vi "CANOpen Refnum to References.vi"(8 "error in (no error)":errorcluster, 11 "CAN Session In":T4) -> (0 "error out":errorcluster, 1 "kill process notifier array":T3, 2 "Write Queue":T1, 3 "Read Queue Array":T1[](array[typedef]), 4 "New Frame Notifier":refnum<notifier>, 5 "CAN Session Queue":T2)   [LabVIEW 2016]
doc: "Extracts the read/write queue references from the CANOpen session refnum."
uses:
  Typedefs/CAN Refnum.ctl
  Typedefs/CAN Session Pointer.ctl
  Typedefs/CAN Communication References.ctl
  Typedefs/kill process notifier array.ctl
  Typedefs/Write Queue.ctl
  Typedefs/FPGA CAN Frame Cluster.ctl
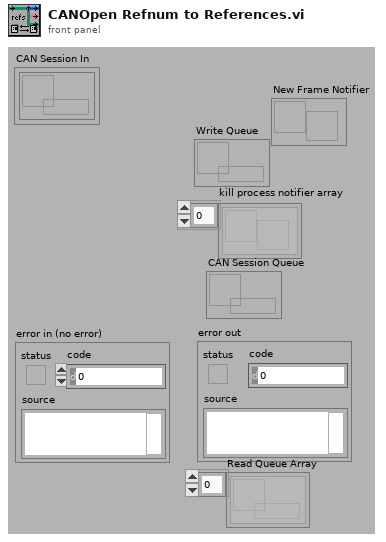
[diagram p1: front panel]
types:
  T1 = typedef "Write Queue.ctl" = refnum<queue>
  T2 = typedef "CAN Session Pointer.ctl" = refnum<queue>
  T3 = typedef "kill process notifier array.ctl" = refnum<notifier>[]
  T4 = typedef "CAN Refnum.ctl" = refnum<k1>
  T5 = typedef "CAN Communication References.ctl" = cluster{"kill process notifier array":T3, "Write Queue":T1, "New Frame Notifier":refnum<notifier>, "Read Queue Array":T1[]}
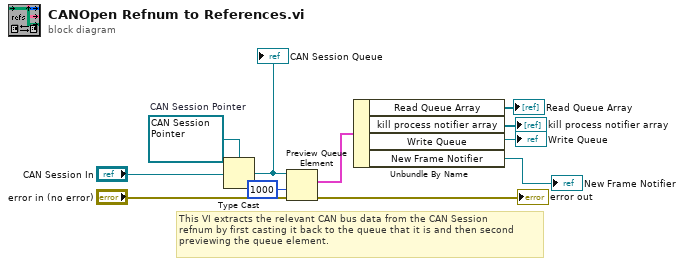
[diagram p0: block diagram]
diagram:
  w11 = T2 refnum  # CAN Session Pointer
  # "This VI extracts the relevant CAN bus data from the CAN Session\nrefnum by first casting it back to the queue that it is and then second\npreviewing the queue element."
  n1 = Type Cast(type=w11, x="CAN Session In") -> (*(type *) &x=w9:T2)
  "CAN Session Queue" <- w9
  n2 = Preview Queue Element(queue=w9, timeout in ms (-1)=1000, error in (no error)="error in (no error)") -> (element=w6:T5, error out=→"error out":errorcluster)  [unwired: 2 out]
  n3 = Unbundle By Name(w6) -> ("Read Queue Array"=→"Read Queue Array":T1[], "kill process notifier array"=→"kill process notifier array":T3, "Write Queue"=→"Write Queue":T1, "New Frame Notifier"=→"New Frame Notifier":refnum<notifier>)
